vi "buildStringTable.vi"(1 "column headers":string[](array[string]), 2 "row headers":string[](array[string]), 3 "text data":string[][](array[string])) -> (0 "output table":string[][](array[string]))   [LabVIEW 2017, in "LabVIEW NPOI.lvlib" / "Document.lvclass"]
uses:
  Document.lvclass
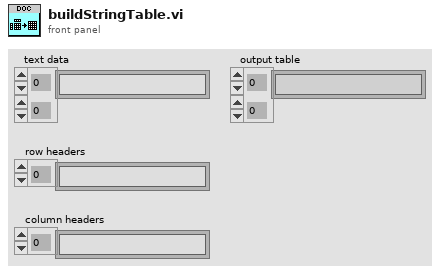
[diagram p1: front panel]
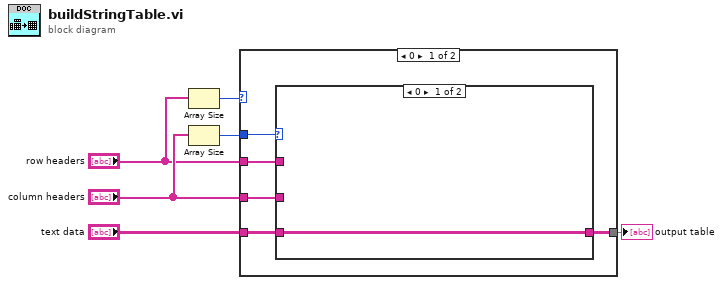
[diagram p0: block diagram]
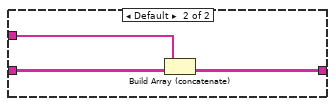
[diagram p2: hidden frame]
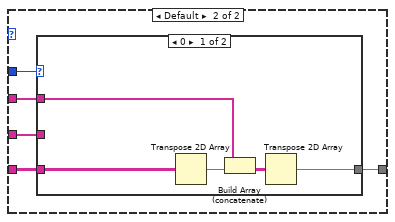
[diagram p3: hidden frame]
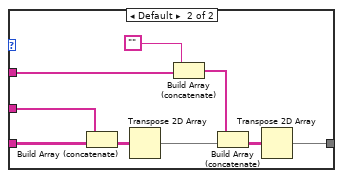
[diagram p4: hidden frame]
diagram:
  n1 = Array Size(array="row headers") -> (size(s)=w1:i32)
  n2 = Array Size(array="column headers") -> (size(s)=w2:i32)
  n3 = case shown="0" w1 {
    tunnel: "text data" -> [w11 w19]
    tunnel: "column headers" -> [w10 w18]
    tunnel: "row headers" -> [w9 w20]
    tunnel: [w8 w16] -> w3
    tunnel: w2 -> [w7 w17]
    frame 0 {
      n4 = case shown="0" w7 {
        tunnel: w10 -> [_ w15]
        tunnel: w11 -> [w12 w14]
        tunnel: [w12 w13] -> w8
        tunnel: w9 -> [_ _]
        frame 0 {
        }
        frame Default {
          n5 = Build Array (concatenate)(w15, w14) -> (w13:string[][])
        }
      }
    }
    frame Default {
      n6 = case shown="0" w17 {
        tunnel: [w22 w32] -> w16
        tunnel: w18 -> [_ w29]
        tunnel: w19 -> [w24 w28]
        tunnel: w20 -> [w25 w26]
        frame 0 {
          n7 = Transpose 2D Array(2D array=w24) -> (transposed array=w23:string[][])
          n8 = Build Array (concatenate)(w25, w23) -> (w21:string[][])
          n9 = Transpose 2D Array(2D array=w21) -> (transposed array=w22:string[][])
        }
        frame Default {
          n10 = Build Array (concatenate)(w29, w28) -> (w27:string[][])
          n11 = Transpose 2D Array(2D array=w27) -> (transposed array=w31:string[][])
          n12 = Build Array (concatenate)("", w26) -> (w30:string[])
          n13 = Build Array (concatenate)(w30, w31) -> (w33:string[][])
          n14 = Transpose 2D Array(2D array=w33) -> (transposed array=w32:string[][])
        }
      }
    }
  }
  "output table" <- w3
